vi "New Data arrived.vi"(8 "error in (no error)":errorcluster caption="错误输入（无错误）", 11 "Data":T1[](array[typedef]) {"Direction" items=["Tx", "Rx"]; "CANType" items=["CAN", "CANFD", "CANFD加速"]}) -> (0 "error out":errorcluster caption="错误输出")   [LabVIEW 2011, in "CAN FD.lvlib"]
uses:
  CAN FD.lvlib
  Typedef/CAN Data.ctl
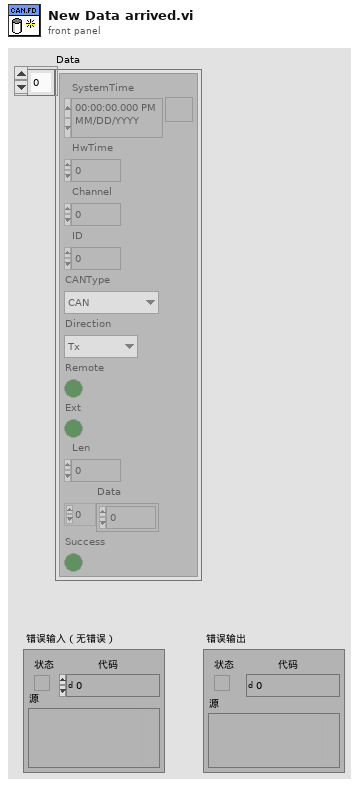
[diagram p1: front panel]
types:
  T1 = typedef "CAN FD.lvlib/CAN Data.ctl" = cluster{"SystemTime":timestamp, "HwTime":dbl, "Channel":u8, "ID":u32, "CANType":i16, "Direction":i16, "Remote":bool, "Ext":bool, "Len":u8, "Data":u8[], "Success":bool}
  T2 = typedef "CAN FD.lvlib/Config.ctl" = cluster{"TimeFormat":u16, "ID Format":u16, "Data Format":u16, "ListLen":u32}
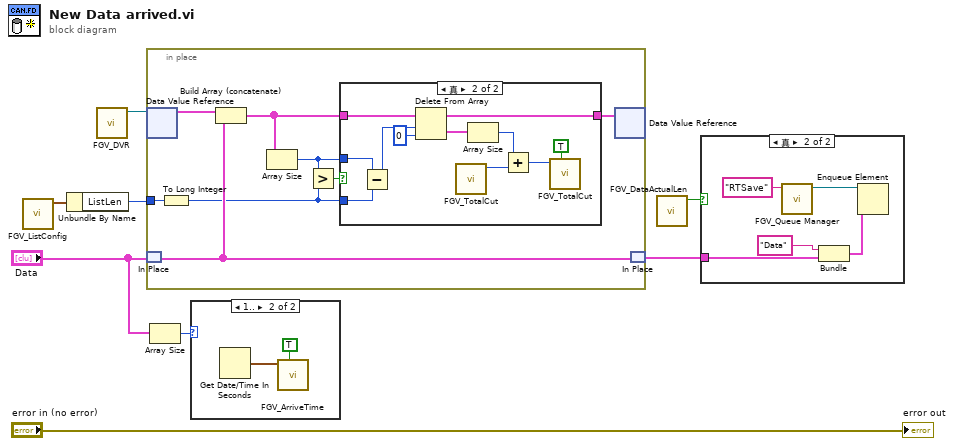
[diagram p0: block diagram]
diagram:
  n1 = call "FGV_ListConfig.vi"() -> ("Config out"=w6:T2)  [unwired: 10 in, 1 out]
  n2 = Unbundle By Name(w6) -> ("ListLen"=w5:u32)
  n3 = call "FGV_DVR.vi"() -> ("DVR"=w7:refnum<data-value>)  [unwired: 10 in, 1 out]
  n4 = in-place {
    in-place-border: w5 -> [w12]
    n5 = in-place-dvr #1(w7) -> (w16:T1[])  [unwired: 1 out]
    n6 = in-place-match #2("Data") -> (w15:T1[])
    n7 = To Long Integer(number=w12) -> (32bit integer=w9:i32)
    n8 = Build Array (concatenate)(w16, w15) -> (w11:T1[])
    n9 = Array Size(array=w11) -> (size(s)=w13:i32)
    n10 = Greater?(x=w13, y=w9) -> (0:w14:bool)
    n11 = case shown="真" w14 {
      tunnel: w13 -> [_ w28]
      tunnel: w9 -> [_ w27]
      tunnel: w11 -> [w17 w26]
      tunnel: [w17 w24] -> w10
      frame False {
      }
      frame True {
        n12 = Subtract(x=w28, y=w27) -> (x-y=w20:i32)
        n13 = Delete From Array(array=w26, length=w20, index=0 ("索引")) -> (deleted portion=w19:T1[], array with subset deleted=w24:T1[])
        n14 = call "FGV_TotalCut.vi"() -> ("Total cut"=w23:i32)  [unwired: 10 in, 1 out]
        n15 = Array Size(array=w19) -> (size(s)=w18:i32)
        n16 = Add(x=w18, y=w23) -> (x+y=w22:i32)
        n17 = call "FGV_TotalCut.vi"("Set"=TRUE, "Total cut"=w22) -> ()  [unwired: 8 in, 2 out]
      }
    }
    n18 = in-place-dvr #1(w10) -> ()  [unwired: 2 out]
    n19 = in-place-match #2(w15) -> (w3:T1[])
  }
  n20 = Array Size(array="Data") -> (size(s)=w1:i32)
  n21 = case shown="1.." w1 {
    frame 0, Default {
    }
    frame 1.. {
      n22 = Get Date/Time In Seconds() -> (seconds since 1Jan1904=w30:timestamp)
      n23 = call "FGV_ArriveTime.vi"("Set"=TRUE, "ArriveTime"=w30) -> ()  [unwired: 8 in, 2 out]
    }
  }
  n24 = call "FGV_DataActualLen.vi"() -> ("RTsave"=w4:bool)  [unwired: 10 in, 1 out]
  n25 = case shown="真" w4 {
    tunnel: w3 -> [_ w33]
    frame False {
    }
    frame True {
      n26 = call "FGV_Queue Manager.vi"("Name"="RTSave") -> ("Queue"=w34:refnum<queue>)  [unwired: 8 in, 2 out]
      n27 = Bundle("Data", "Data"=w33) -> (w32:cluster{string, "Data":T1[]})  [unwired: 1 in]
      n28 = Enqueue Element(queue=w34, element=w32) -> ()  [unwired: 2 in, 3 out]
    }
  }
  "error out" <- "error in (no error)"
